vi "lissagu.vi"() -> ()   [LabVIEW 2021]
panel:
  in  "stop":bool
  in  "Knob":dbl(knob) scale=0.0..90.0
  out "XY Graph":cluster{dbl[], dbl[]}(graph)
  in  "enter freq a2":dbl
  in  "enter freq a1":dbl
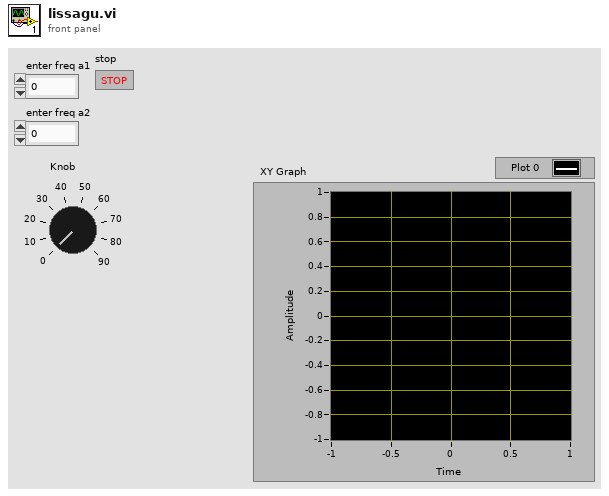
[diagram p1: front panel]
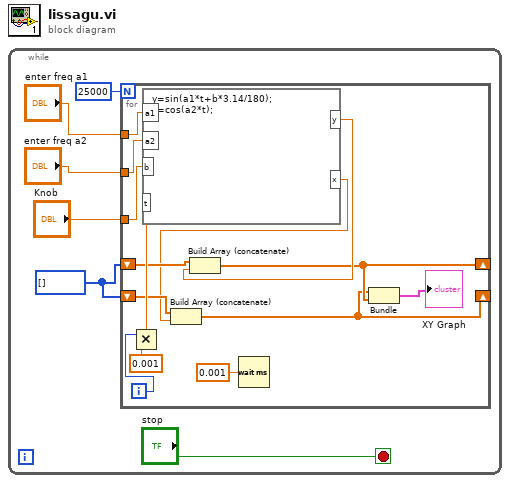
[diagram p0: block diagram]
diagram:
  n1 = while {
    stop <- "stop" stop-if-true
    w5 = i32[] []
    n2 = for {
      N: 25000 -> [_]
      shift-right: [w13] -> _
      shift-left: w5 -> [w17]
      shift-right: [w12] -> _
      shift-left: w5 -> [w16]
      tunnel: "enter freq a1" -> [w10]
      tunnel: "Knob" -> [w9]
      tunnel: "enter freq a2" -> [w8]
      i -> [w19]
      n3 = Multiply(x=w19, y=0.001) -> (x*y=w18:dbl)
      n4 = formula code="y=sin(a1*t+b*3.14/180);\nx=cos(a2*t);"("a1"=w10, "a2"=w8, "b"=w9, "t"=w18) -> ("y"=w14:dbl, "x"=w15:dbl)
      n5 = Build Array (concatenate)(w16, w15) -> (w12:dbl[])
      n6 = Build Array (concatenate)(w17, w14) -> (w13:dbl[])
      n7 = Wait (ms)(milliseconds to wait=0.001) -> ()  [unwired: 1 out]
      n8 = Bundle(w12, w13) -> (→"XY Graph":cluster{dbl[], dbl[]})  [unwired: 1 in]
    }
  }
